vi "CRYSelect waveform by name.vi"(9 "Wave name desired (just name, if flat wave not wired)":string, 10 "Wave name desired (flat Wave)":string, 11 "Waveform Array":T2 {"Y dB ref" format="%.1f"; "Y axis" items=["Log", "Lin"]; "Y data" items=["dB", "Lin"]; "X data" items=["dB", "Lin"]}) -> (0 "Exists?":bool, 1 "Valid curve desired?":bool, 3 "Desired Waveform":T1={"Waveform"={"X0"=0.0, "dX"=0.0, "Y"=[]}, "X data"=1, "Y data"=1, "Y axis"=1, "X unit"="s", "Y unit"="V", "Y dB ref"=1.0, "display Y"=TRUE, "display X"=TRUE, "Overload?"=FALSE, "Test Info"="", "Step No."=0, "Name"="", "protected"=FALSE, "Sqc history"=[], "Signal Channel ID"=0, "Plot Settings"={"Color"=0, "Interpolation"=0, "Point Style"=0, "Line Style"=0, "Point Color"=0, "Line Width"=0, "Bar Plot Style"=0, "Fill To"=0}, "AutoProtect"=FALSE} {"Y dB ref" format="%.1f"; "Y axis" items=["Log", "Lin"]; "Y data" items=["dB", "Lin"]; "X data" items=["dB", "Lin"]}, 5 "index of element":i32)   [LabVIEW 2013]
uses:
  Typedef Control/CRYWaveform Cluster Array.ctl
  Typedef Control/CRYWaveform Cluster.ctl
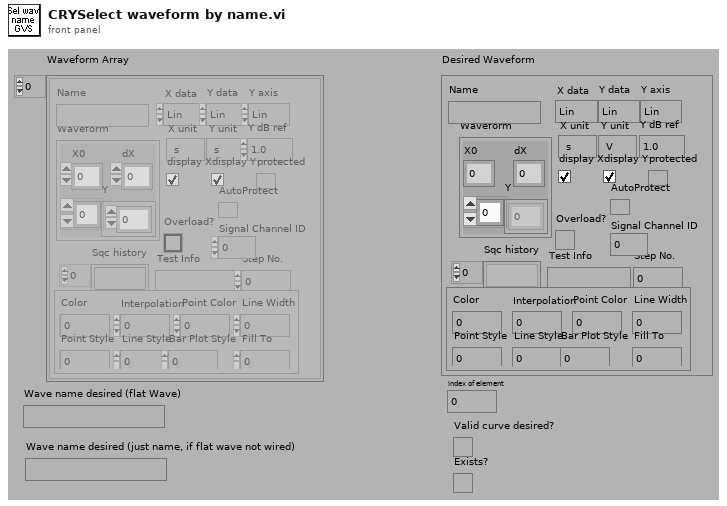
[diagram p1: front panel]
types:
  T1 = typedef "CRYWaveform Cluster.ctl" = cluster{"Waveform":cluster{"X0":dbl, "dX":dbl, "Y":sgl[]}, "X data":u16, "Y data":u16, "Y axis":u16, "X unit":string, "Y unit":string, "Y dB ref":dbl, "display Y":bool, "display X":bool, "Overload?":bool, "Test Info":string, "Step No.":i32, "Name":string, "protected":bool, "Sqc history":string[], "Signal Channel ID":i32, "Plot Settings":cluster{"Color":u32, "Interpolation":u8, "Point Style":u8, "Line Style":u8, "Point Color":u32, "Line Width":u8, "Bar Plot Style":u8, "Fill To":i16}, "AutoProtect":bool}
  T2 = typedef "CRYWaveform Cluster Array.ctl" = T1[]
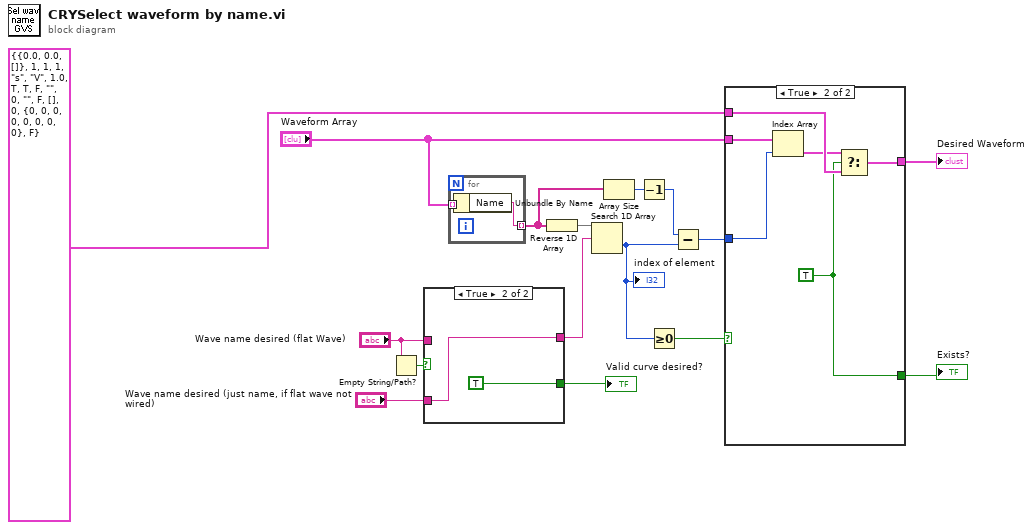
[diagram p0: block diagram]
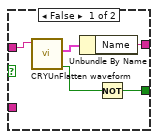
[diagram p2: hidden frame]
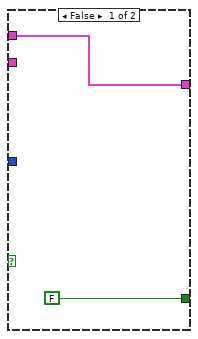
[diagram p3: hidden frame]
diagram:
  n1 = Empty String/Path?(string/path="Wave name desired (flat Wave)") -> (empty?=w5:bool)
  n2 = case shown="True" w5 {
    tunnel: "Wave name desired (flat Wave)" -> [w19 _]
    tunnel: [w21 w23] -> w10
    tunnel: [w20 TRUE] -> w7
    tunnel: "Wave name desired (just name, if flat wave not wired)" -> [_ w23]
    frame False {
      n3 = call "CRYUnFlatten waveform.vi"("Unflatten Waveform"=w19) -> ("Error?"=w17:bool, "Waveform Cluster"=w18:T1)  [unwired: 8 in, 1 out]
      n4 = Unbundle By Name(w18) -> ("Name"=w21:string)
      n5 = Not(x=w17) -> (.not. x?=w20:bool)
    }
    frame True {
    }
  }
  "Valid curve desired?" <- w7
  n6 = for {
    tunnel: "Waveform Array" -> [w25] mode=indexing
    tunnel: [w24] -> w14 mode=indexing
    n7 = Unbundle By Name(w25) -> ("Name"=w24:string)
  }
  n8 = Reverse 1D Array(array=w14) -> (reversed array=w16:string[])
  n9 = Search 1D Array(1D array=w16, element=w10) -> (index of element=w11:i32)  [unwired: 1 out]
  "index of element" <- w11
  n10 = Array Size(array=w14) -> (size(s)=w13:i32)
  n11 = Decrement(x=w13) -> (x-1=w12:i32)
  n12 = Greater Or Equal To 0?(x=w11) -> (x >= 0?=w9:bool)
  n13 = Subtract(x=w12, y=w11) -> (x-y=w15:i32)
  n14 = case shown="True" w9 {
    tunnel: "Waveform Array" -> [_ w33]
    tunnel: w15 -> [_ w32]
    tunnel: [w26 w30] -> w1
    tunnel: T1 {"Waveform"={"X0"=0.0, "dX"=0.0, "Y"=[]}, "X data"=1, "Y data"=1, "Y axis"=1, "X unit"="s", "Y unit"="V", "Y dB ref"=1.0, "display Y"=TRUE, "display X"=TRUE, "Overload?"=FALSE, "Test Info"="", "Step No."=0, "Name"="", "protected"=FALSE, "Sqc history"=[], "Signal Channel ID"=0, "Plot Settings"={"Color"=0, "Interpolation"=0, "Point Style"=0, "Line Style"=0, "Point Color"=0, "Line Width"=0, "Bar Plot Style"=0, "Fill To"=0}, "AutoProtect"=FALSE} ("Desired Waveform") -> [w26 w31]
    tunnel: [FALSE w29] -> w8
    frame False {
    }
    frame True {
      w29 = TRUE
      n15 = Index Array(array=w33, index=w32) -> (element=w28:T1)
      n16 = Select(t=w28, s=w29, f=w31) -> (s? t:f=w30:T1)
    }
  }
  "Exists?" <- w8
  "Desired Waveform" <- w1
